vi "Generate Patch Sequence Images.vi"(4 "Green":path[](array[path]), 5 "Red":path[](array[path]), 6 "Predominant ROI type":T1=enum."Comp. volume", 7 "Imaging Protocol":T2=enum."Live Imaging", 8 "error in (no error)":errorcluster, 9 "Green TIFF handles":i32[](array[numeric]), 10 "Red TIFF handles":i32[](array[numeric]), 11 "TDMS file path & name":path) -> (0 "error out":errorcluster, 2 "Destination fiolder":path)   [LabVIEW 2017]
uses:
  Typedefs/Imaging Protocols enum.ctl
  Typedefs/ROI ID Enum.ctl
  User Interface/Visualisation/Functional Imaging Viewer/SubVIs/Experiment header interface/Typedefs/Header file sections.ctl
  User Interface/Visualisation/Functional Imaging Viewer/SubVIs/Experiment header interface/Typedefs/Header file actions.ctl
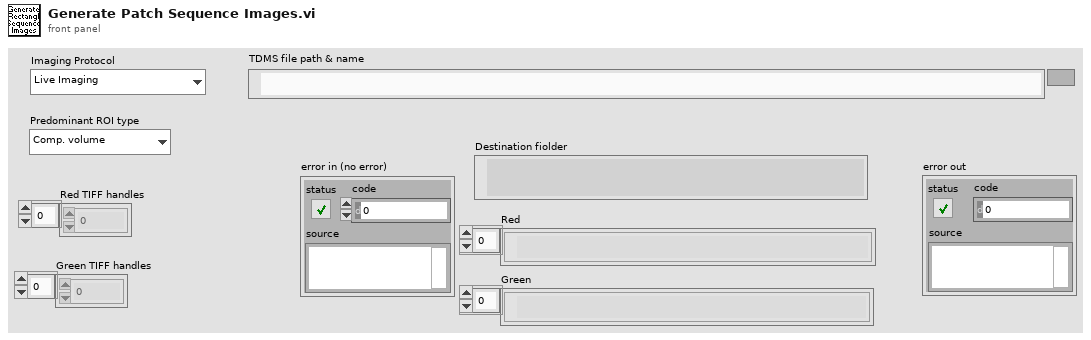
[diagram p1: front panel]
types:
  T1 = typedef "ROI ID Enum.ctl" = enum16{"Point", "MiniScan", "Comp. MiniScan", "Rectangle", "Comp. volume", "Arb. plane point"}
  T2 = typedef "Imaging Protocols enum.ctl" = enum16{"AOL Z-Stack", "Motor Z Stack", "Functional Acquisition", "Single Plane Acquisition", "Volume Acquisition", "Live Imaging", "Live Plane Imaging", "Live Volume Imaging"}
  T3 = typedef "Header file actions.ctl" = enum16{"Create", "Open", "Read All", "Read Section", "Write All", "Write Section", "Close"}
  T4 = typedef "Header file sections.ctl" = enum16{"ALL SECTIONS", "LOGIN", "GLOBAL PARAMETERS", "IMAGING MODES", "TIME SERIES", "MOTOR Z-STACK", "AOL Z-STACK", "FUNCTIONAL IMAGING", "MOVEMENT CORRECTION", "CALIBRATION", "STATISTICS", "BIOLOGY INFORMATION"}
  T5 = typedef "Header parameters cluster-ALL.ctl" = cluster{"LOGIN":T6, "GLOBAL PARAMETERS":T7, "IMAGING MODES":T9, "TIME SERIES":T10, "MOTOR Z-STACK ":T13, "AOL Z-STACK":T14, "FUNCTIONAL IMAGING":T15, "MOVEMENT CORRECTION":T19, "CALIBRATION":T21, "STATISTICS":T22, "BIOLOGY INFORMATION":T23}
  T6 = typedef "Header params -Login.ctl" = cluster{"User":string, "Profile":string, "Software Version":string, "Experiment Date Time":timestamp}
  T7 = typedef "Header params-Global Parameters.ctl" = cluster{"MicroscopeID":string, "Microscope Type":string, "Objective":string, "Field of View (um)":dbl, "Fill time (us)":dbl, "Experiment Type":T8, "Stimuli Trigger":bool, "Speed Logging":bool}
  T8 = typedef "Experiment Type.ctl" = enum16{"In vivo", "In vitro", "Testing", "Calibration", "Other"}
  T9 = typedef "Header params-Imaging Modes.ctl" = cluster{"Time Series":bool, "Motor Zstack":bool, "AOL Zstack":bool, "Functional Imaging":bool}
  T10 = typedef "Header params-Time Series.ctl" = cluster{"Basic Image meta data":T11, "AOL z":dbl}
  T11 = typedef "Header params-Basic image meta data.ctl" = cluster{"Wavelength (nm)":dbl, "# averaged frames":dbl, "laser power (%)":dbl, "Pockels":dbl, "pixel dwell time (us)":dbl, "pmt 1":dbl, "pmt 2":dbl, "back apperture":dbl, "zoom":dbl, "field of view":dbl, "Frame Size":T12, "AOL x centre":dbl, "AOL y centre":dbl, "Stage x position":dbl, "Stage y position":dbl, "Stage z position":dbl}
  T12 = typedef "Frame Size.ctl" = u16
  T13 = typedef "Header params-Motor Z-stack.ctl" = cluster{"Hdr Basic Image meta data":T11, "Z Start":dbl, "Z Stop":dbl, "No of Planes":i32}
  T14 = typedef "Header params-AOL Z-stack.ctl" = cluster{"Hdr Basic Image meta data":T11, "Z Start":dbl, "Z Stop":dbl, "No of Planes":i32}
  T15 = typedef "Header params-Functional Imaging.ctl" = cluster{"Functional Mode":T16, "Pockels Modulation":bool, "Number of pois":dbl, "Number of miniscans":dbl, "Number of cycles":dbl, "Number of trials":dbl, "Miniscan dwell time per pixel (us)":dbl, "Number of pixels in miniscan":dbl, "poi dwell time":dbl, "Rectangle ROI length":dbl, "Rectangle ROI height":dbl, "AOL Mode":T17, "Plane Mode":T18, "video length (sec)":dbl, "Frame rate (fps)":dbl, "Stimuli Timing (usec)":dbl, "Acquisition Length":dbl, "Basic Image meta data":T11, "Z Start (um)":dbl, "Z Stop (um)":dbl}
  T16 = typedef "Functional Mode.ctl" = enum16{"Point", "Line", "Patch", "Plane", "Volume"}
  T17 = typedef "AOL modes.ctl" = enum16{"Raster", "Structural", "Pointing", "Mini Scan", "Alignment"}
  T18 = typedef "Plane Mode.ctl" = u16
  T19 = typedef "Header params-Movement correction.ctl" = cluster{"Movement Correction":bool, "Axial Reference":bool, "Reference X Pixels":dbl, "Reference Y Pixels":dbl, "Reference Source":T20, "Reference dwell time (us)":dbl, "Number of Z lines":dbl, "Size of Z pixels":dbl, "Axial Pixels":dbl, "Reference Zoom":dbl, "Reference Average":dbl, "Proportional Scale":dbl, "Integral Scale":dbl, "Proportional Scale Z":dbl, "Integral Scale Z":dbl, "Scan Interval":dbl, "Ref Plot Refresh Rate":dbl}
  T20 = typedef "Reference source.ctl" = enum16{"Green channel", "Red channel"}
  T21 = typedef "Header params-Calibration Setup.ctl" = cluster{"Pockels Calibration File":path, "Calibration_ini file":path, "Setup_ini file":path}
  T22 = typedef "Header params-statistics.ctl" = cluster{"Z-stack duration (sec)":dbl, "Number of acquired data-points":dbl, "Acquisition time (ms)":dbl, "Number of acquired frames":dbl}
  T23 = typedef "Biology Information.ctl" = cluster{"Animal Code or Name":string, "Animal DoB":string, "Animal Age":string, "Animal Sex":string, "Animal Weight":string, "Date of Injection":string, "Date of Implant":string, "Site of Injection":string, "Animal Ear Notch":string, "AAV constructs":string, "Genetic background":string, "Optical reporter":string, "Region of brain imaged":string, "Other \ncomments":string}
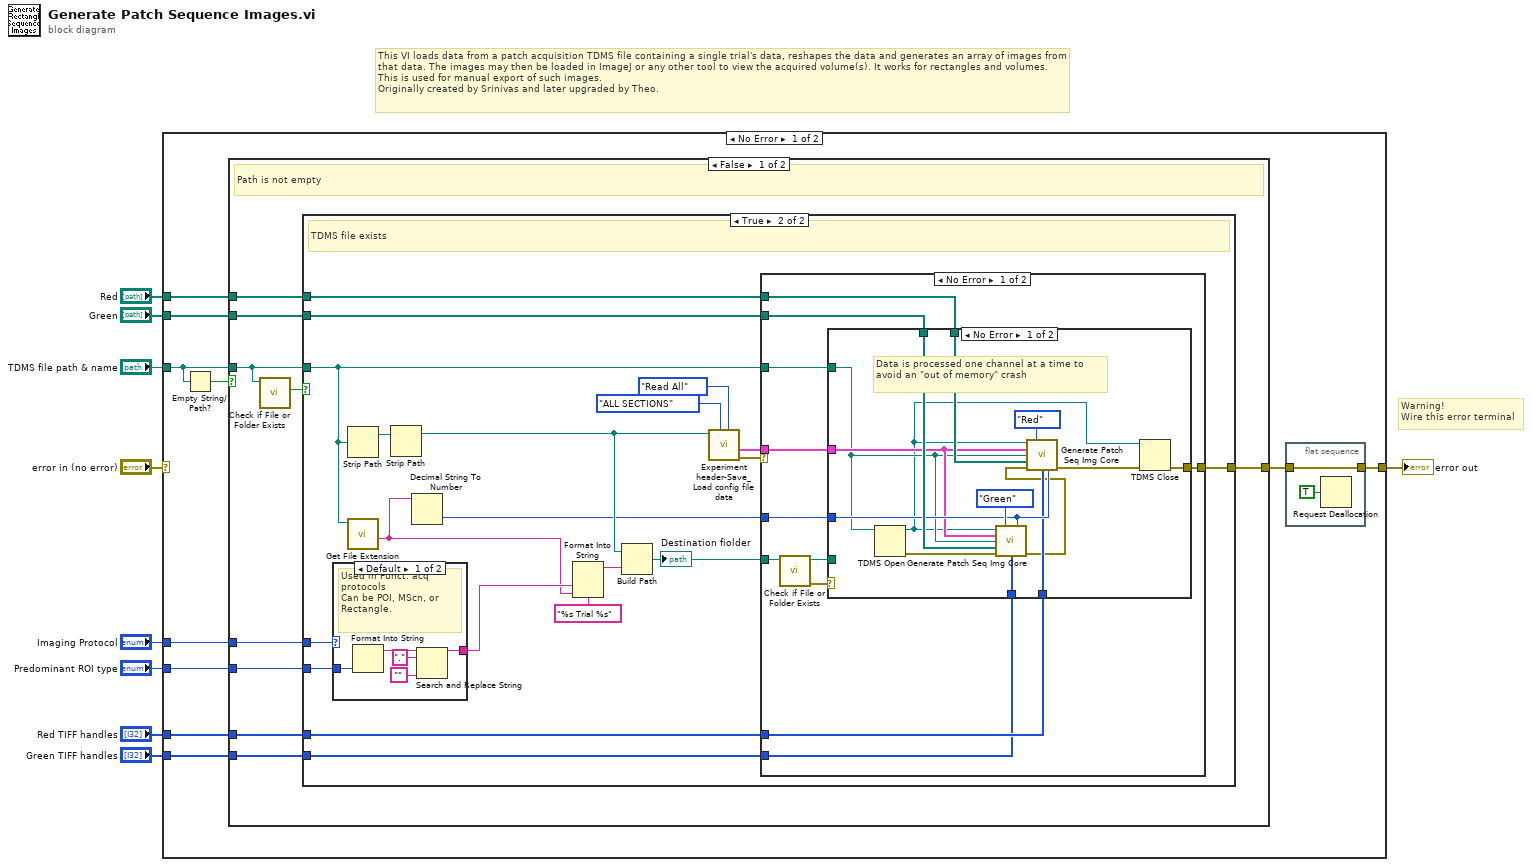
[diagram p0: block diagram]
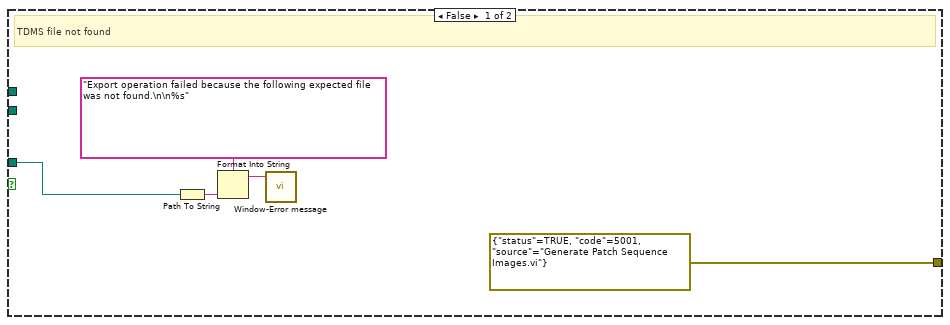
[diagram p2: hidden frame]
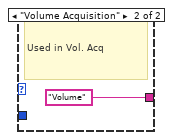
[diagram p5: hidden frame]
diagram:
  # "This VI loads data from a patch acquisition TDMS file containing a single trial's data, reshapes the data and generates an array of images from that data. The images may then be loaded in ImageJ or any other tool to view the acquired volume(s). It works for rectangles and volumes. This is used for manual export of such images.\nOriginally created by Srinivas and later upgraded by Theo."
  # "Warning!\nWire this error terminal"
  n1 = case shown="No Error" "error in (no error)" {
    selector: "error in (no error)" -> [_ w88]
    tunnel: "TDMS file path & name" -> [w18 _]
    tunnel: "Imaging Protocol" -> [w17 _]
    tunnel: "Predominant ROI type" -> [w16 _]
    tunnel: "Green" -> [w14 _]
    tunnel: "Red" -> [w13 _]
    tunnel: "Red TIFF handles" -> [w12 _]
    tunnel: "Green TIFF handles" -> [w11 _]
    tunnel: [w10 w88] -> w2
    frame No Error {
      n2 = Empty String/Path?(string/path=w18) -> (empty?=w19:bool)
      n3 = case shown="False" w19 {
        tunnel: w18 -> [w29 _]
        tunnel: [w28 _] -> w15
        tunnel: w17 -> [w27 _]
        tunnel: w16 -> [w26 _]
        tunnel: w14 -> [w25 _]
        tunnel: w13 -> [w24 _]
        tunnel: w12 -> [w23 _]
        tunnel: w11 -> [w22 _]
        frame False {
          # "Path is not empty"
          n4 = call <vilib>:"Check if File or Folder Exists.vi"("path"=w29) -> ("file or folder exists?"=w30:bool)  [unwired: 8 in, 2 out]
          n5 = case shown="True" w30 {
            tunnel: w29 -> [w34 w55]
            tunnel: [errorcluster {"status"=TRUE, "code"=5001, "source"="Generate Patch Sequence Images.vi"} ("error IO") w53] -> w28
            tunnel: w27 -> [_ w51]
            tunnel: w26 -> [_ w50]
            tunnel: w25 -> [_ w49]
            tunnel: w24 -> [_ w48]
            tunnel: w23 -> [_ w39]
            tunnel: w22 -> [_ w38]
            frame False {
              # "TDMS file not found"
              n6 = Path To String(path=w34) -> (string=w33:string)
              n7 = Format Into String(format string="Export operation failed because the following expected file was not found.\n\n%s", w33) -> (resulting string=w32:string)  [unwired: 2 in, 1 out]
              n8 = call "Window-Error message.vi"("Message"=w32) -> ()  [unwired: 10 in, 1 out]
            }
            frame True {
              # "TDMS file exists"
              n9 = case shown="Default" w51 {
                tunnel: w50 -> [w86 _]
                tunnel: [w82 "Volume" ("result string")] -> w44
                frame Default {
                  # "Used in Funct. acq protocols\nCan be POI, MScn, or Rectangle."
                  n10 = Format Into String(w86) -> (resulting string=w85:string)  [unwired: 3 in, 1 out]
                  n11 = Search and Replace String(input string=w85, search string=".", replace string="" ("replace string (\"\")")) -> (result string=w82:string)  [unwired: 5 in, 3 out]
                }
                frame "Volume Acquisition" {
                  # "Used in Vol. Acq"
                }
              }
              n12 = Strip Path(path=w55) -> (stripped path=w46:path)  [unwired: 1 out]
              n13 = call <vilib>:"Get File Extension.vi"("file"=w55) -> ("filename without extension"=w42:string)  [unwired: 6 in, 4 out]
              n14 = Strip Path(path=w46) -> (stripped path=w54:path)  [unwired: 1 out]
              n15 = Decimal String To Number(string=w42) -> (number=w47:i32)  [unwired: 2 in, 1 out]
              n16 = Format Into String(format string="%s Trial %s", w44, w42) -> (resulting string=w43:string)  [unwired: 2 in, 1 out]
              n17 = Build Path(base path=w54, name or relative path=w43) -> (appended path=w52:path)
              "Destination fiolder" <- w52
              n18 = call "Experiment header-Save_Load config file data.vi"("Header file actions"=Header_file_actions."Read All", "Header file sections"=Header_file_sections."ALL SECTIONS", "Experiment data folder path"=w54) -> ("error out"=w40:errorcluster, "All header parameters out"=w41:T5)  [unwired: 7 in]
              n19 = case shown="No Error" w40 {
                tunnel: w52 -> [w66 _]
                tunnel: w55 -> [w65 _]
                tunnel: w41 -> [w63 _]
                tunnel: [w64 _] -> w53
                tunnel: w49 -> [w62 _]
                tunnel: w48 -> [w61 _]
                tunnel: w47 -> [w60 _]
                tunnel: w39 -> [w57 _]
                tunnel: w38 -> [w56 _]
                frame No Error {
                  n20 = call <vilib>:"Check if File or Folder Exists.vi"("path"=w66) -> ("error out"=w58:errorcluster, "dup path"=w59:path)  [unwired: 8 in, 1 out]
                  n21 = case shown="No Error" w58 {
                    selector: w58 -> [_ w81]
                    tunnel: w59 -> [_ _]
                    tunnel: w65 -> [w71 _]
                    tunnel: w63 -> [w72 _]
                    tunnel: [w76 w81] -> w64
                    tunnel: w62 -> [w79 _]
                    tunnel: w61 -> [w78 _]
                    tunnel: w60 -> [w77 _]
                    tunnel: w57 -> [w75 _]
                    tunnel: w56 -> [w74 _]
                    frame No Error {
                      # "Data is processed one channel at a time to avoid an \"out of memory\" crash"
                      n22 = TDMS Open(11:w71) -> (0:w70:errorcluster, 3:w69:refnum<k34>)  [unwired: 6 in]
                      n23 = call "Generate Patch Seq Img Core.vi"("tdms file ref"=w69, "Channel to process"=enum16{"Red", "Green"}."Green", "All header parameters"=w72, "TDMS file path & name"=w71, "Patch Image Folder"=w79, "error in (no error)"=w70, "TIFF file handles"=w74, "Trial Number"=w77) -> ("error out"=w68:errorcluster)  [unwired: 6 in, 1 out]
                      n24 = call "Generate Patch Seq Img Core.vi"("tdms file ref"=w69, "Channel to process"=enum16{"Red", "Green"}."Red", "All header parameters"=w72, "TDMS file path & name"=w71, "Patch Image Folder"=w78, "error in (no error)"=w68, "TIFF file handles"=w75, "Trial Number"=w77) -> ("error out"=w67:errorcluster)  [unwired: 6 in, 1 out]
                      n25 = TDMS Close(8:w67, 11:w69) -> (0:w76:errorcluster)  [unwired: 1 out]
                    }
                    frame Error {
                    }
                  }
                }
                frame Error {
                  # "Error reporting handled inside the subVI."
                }
              }
            }
          }
        }
        frame True {
          # "Path is empty"
        }
      }
      n26 = flat-sequence {
        tunnel: w15 -> [w20]
        tunnel: [w20] -> w10
        frame #0 {
          n27 = Request Deallocation(TRUE ("flag")) -> ()
        }
      }
    }
    frame Error {
    }
  }
  "error out" <- w2
